vi "SDCP Receiver and Transmitter - Rx Base.vi"(1 "error in (no error)":errorcluster) -> (0 "error out":errorcluster)   [LabVIEW 2020]
uses:
  Typedefs/SDCP - Serial Port Control - Commands.ctl
  Typedefs/SDCP SMF logger - SMF with timestamp.ctl
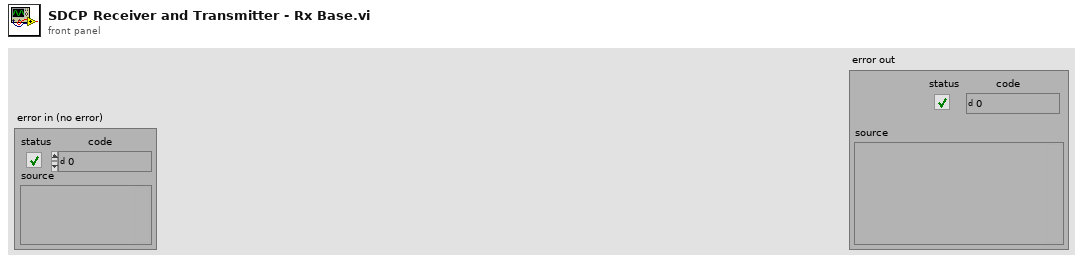
[diagram p1: front panel]
types:
  T1 = typedef "SDCP - Serial Port Control - Commands.ctl" = enum16{"Open", "Read", "Write", "Get instance", "Close"}
  T2 = typedef "SDCP SMF Receiver and Transmitter - Notifier and Queues.ctl" = cluster{"Trace Queue":refnum<queue>, "Tx - Log Table Queue":refnum<queue>, "Tx - User Queue":refnum<queue>, "Rx - Log Table Queue":refnum<queue>, "Rx - User Queue":refnum<queue>, "Log status Notifier":refnum<notifier>, "Plot Queue":refnum<queue>}
  T3 = typedef "SDCP SMF logger - SMF with timestamp.ctl" = cluster{"Bytes":u8[], "Checksum":bool, "Time (ms)":u32, "Tx/Rx":string}
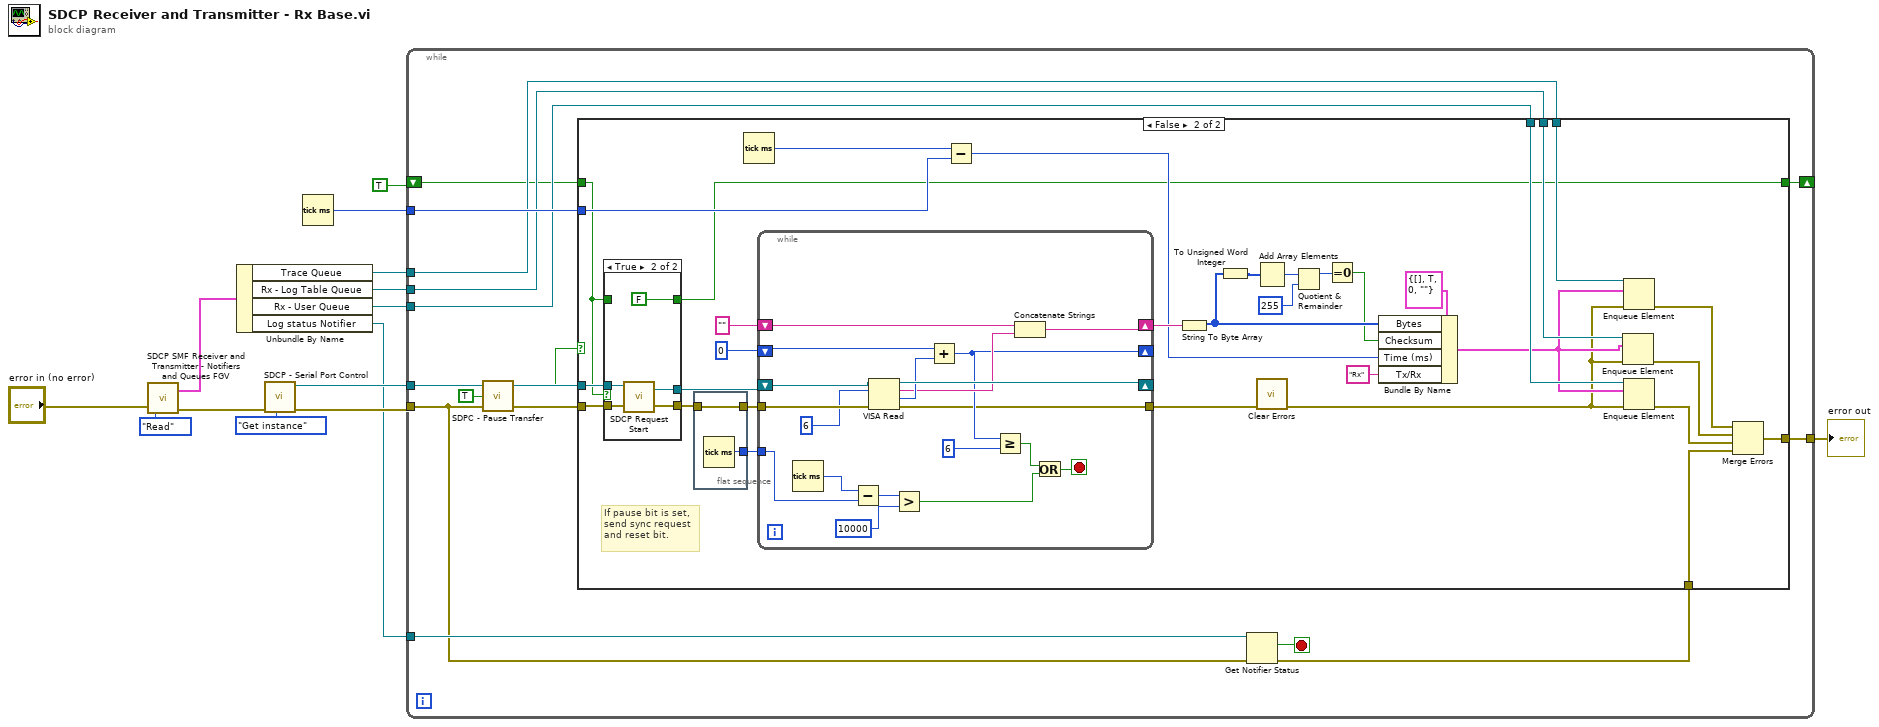
[diagram p0: block diagram]
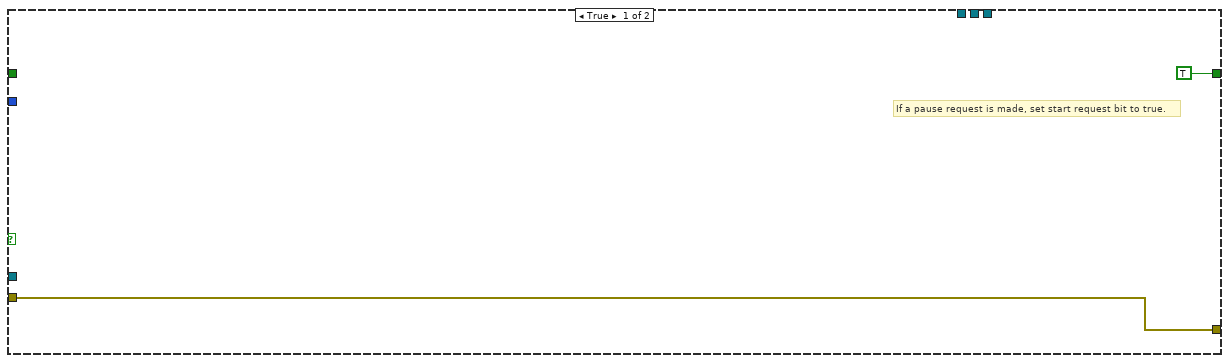
[diagram p2: hidden frame]
diagram:
  n1 = call "SDCP SMF Receiver and Transmitter - Notifiers and Queues FGV.vi"("error in (no error)"="error in (no error)", "Command"=enum16{"Initialize", "Read", "Deinitialize"}."Read") -> ("error out"=w7:errorcluster, "Output"=w12:T2)
  n2 = Unbundle By Name(w12) -> ("Trace Queue"=w11:refnum<queue>, "Rx - Log Table Queue"=w10:refnum<queue>, "Rx - User Queue"=w9:refnum<queue>, "Log status Notifier"=w3:refnum<notifier>)
  n3 = call "SDCP - Serial Port Control.vi"("Command"=SDCP_-_Serial_Port_Control_-_Commands."Get instance", "error in (no error)"=w7) -> ("error out"=w6:errorcluster, "VISA out"=w4:refnum<visa-resource-name>)  [unwired: 6 in, 2 out]
  n4 = Tick Count (ms)() -> (millisecond timer value=w8:u32)
  n5 = while {
    tunnel: w6 -> [w20]
    tunnel: w11 -> [w25]
    tunnel: w10 -> [w24]
    tunnel: w9 -> [w23]
    tunnel: w8 -> [w26]
    tunnel: w4 -> [w29]
    tunnel: w3 -> [w28]
    tunnel: [w21] -> w2
    shift-right: [w15] -> _
    shift-left: TRUE -> [w16]
    stop <- w27 stop-if-true
    n6 = call "SDPC - Pause Transfer.vi"("error in (no error)"=w20, "RD/nWR"=TRUE) -> ("error out"=w19:errorcluster, "Transfer paused"=w18:bool)  [unwired: 2 in]
    n7 = Get Notifier Status(notifier=w28, error in (no error)=w20) -> (current notification=w27:bool, error out=w22:errorcluster)  [unwired: 3 out]
    n8 = case shown="False" w18 {
      tunnel: w29 -> [_ w36]
      tunnel: w26 -> [_ w53]
      tunnel: w25 -> [_ w49]
      tunnel: w24 -> [_ w48]
      tunnel: w23 -> [_ w47]
      tunnel: w22 -> [_ w42]
      tunnel: [w31 w41] -> w21
      tunnel: w19 -> [w31 w37]
      tunnel: w16 -> [_ w33]
      tunnel: [TRUE w32] -> w15
      frame True {
        # "If a pause request is made, set start request bit to true."
      }
      frame False {
        # "If pause bit is set,\nsend sync request\nand reset bit."
        n9 = case shown="True" w33 {
          tunnel: w37 -> [w66 w72]
          tunnel: w36 -> [w67 w71]
          tunnel: [w67 w70] -> w35
          tunnel: [w66 w69] -> w34
          tunnel: [w65 FALSE] -> w32
          tunnel: w33 -> [w65 _]
          frame False {
          }
          frame True {
            n10 = call "SDCP Request Start.vi"("error in (no error)"=w72, "COM Port"=w71) -> ("error out"=w69:errorcluster, "COM Port Out"=w70:refnum<visa-resource-name>)
          }
        }
        n11 = flat-sequence {
          tunnel: w34 -> [w74]
          tunnel: [w74] -> w39
          tunnel: [w73] -> w38
          frame #0 {
            n12 = Tick Count (ms)() -> (millisecond timer value=w73:u32)
          }
        }
        n13 = Tick Count (ms)() -> (millisecond timer value=w54:u32)
        n14 = while {
          tunnel: w39 -> [w93]
          shift-right: [w84] -> w62
          shift-left: "" -> [w86]
          shift-right: [w83] -> _
          shift-left: 0 -> [w89]
          shift-right: [w90] -> _
          shift-left: w35 -> [w92]
          tunnel: [w82] -> w50
          tunnel: w38 -> [w80]
          stop <- w77 stop-if-true
          n15 = Tick Count (ms)() -> (millisecond timer value=w81:u32)
          n16 = Subtract(x=w81, y=w80) -> (x-y=w79:u32)
          n17 = VISA Read(VISA resource name=w92, byte count=u32 6, error in (no error)=w93) -> (VISA resource name out=w90:refnum<visa-resource-name>, read buffer=w85:string, return count=w88:u32, error out=w82:errorcluster)
          n18 = Greater?(x=w79, y=u32 10000) -> (0:w75:bool)
          n19 = Add(x=w89, y=w88) -> (x+y=w83:u32)
          n20 = Greater Or Equal?(x=w83, y=u32 6) -> (x >= y?=w76:bool)
          n21 = Concatenate Strings(w86, w85) -> (w84:string)
          n22 = Or(x=w76, y=w75) -> (x .or. y?=w77:bool)
        }
        n23 = Subtract(x=w54, y=w53) -> (x-y=w52:u32)
        n24 = String To Byte Array(string=w62) -> (unsigned byte array=w60:u8[])
        n25 = To Unsigned Word Integer(number=w60) -> (unsigned 16bit integer=w59:u16[])
        n26 = Add Array Elements(numeric array=w59) -> (sum=w58:u16)
        n27 = call <vilib>:"Clear Errors.vi"("error in (no error)"=w50) -> ("error out"=w40:errorcluster)  [unwired: 5 in, 1 out]
        n28 = Quotient & Remainder(x=w58, y=u16 255) -> (x-y*floor(x/y)=w56:u16)  [unwired: 1 out]
        n29 = Equal To 0?(x=w56) -> (x = 0?=w55:bool)
        n30 = Bundle By Name(cluster=T3 {"Bytes"=[], "Checksum"=TRUE, "Time (ms)"=0, "Tx/Rx"=""} ("SMF with timestamp"), "Bytes"=w60, "Checksum"=w55, "Time (ms)"=w52, "Tx/Rx"="Rx") -> (w46:T3)
        n31 = Enqueue Element(queue=w48, element=w46, error in (no error)=w40) -> (error out=w44:errorcluster)  [unwired: 1 in, 2 out]
        n32 = Enqueue Element(queue=w49, element=w46, error in (no error)=w40) -> (error out=w45:errorcluster)  [unwired: 1 in, 2 out]
        n33 = Enqueue Element(queue=w47, element=w46, error in (no error)=w40) -> (error out=w43:errorcluster)  [unwired: 1 in, 2 out]
        n34 = Merge Errors(w45, w44, w43, w42) -> (w41:errorcluster)
      }
    }
  }
  "error out" <- w2
